vi "Progress bar v2.vi"(7 "TIme (s)":dbl=10.0, 8 "error in":errorcluster, 11 "Title":string="Preparing GUI") -> (0 "error out":errorcluster)   [LabVIEW 2021]
uses:
  <vilib>/NI/Progress Bar/Controls/Update Bar Actions.ctl
  <vilib>/NI/Progress Bar/Controls/Progress Bar Properties.ctl
  f8578292-8b37-437c-93d2-4d8660ecfccc.vi
  114d9f00-15c4-4ec7-b9fc-572f42474f64.vi
  911e5ed0-5c28-4744-8a2b-9f7e262dfa91.vi
  eb646fbe-3ace-4864-911c-cb9f93faacb5.vi
  875ffc95-6fd8-47bf-be2f-a53a9a05b130.vi
  8d024e92-ce25-45d8-b0eb-876bcb212ffe.vi
  0a453649-e7a0-4eaf-b47a-dfd7043e0d01.vi
  be3f16ba-4c0f-4040-8c78-39f5a151251f.vi
  12f81415-701e-4c93-8868-a36497b1982f.vi
  <vilib>/NI/Progress Bar/Progress Bar.lvlib
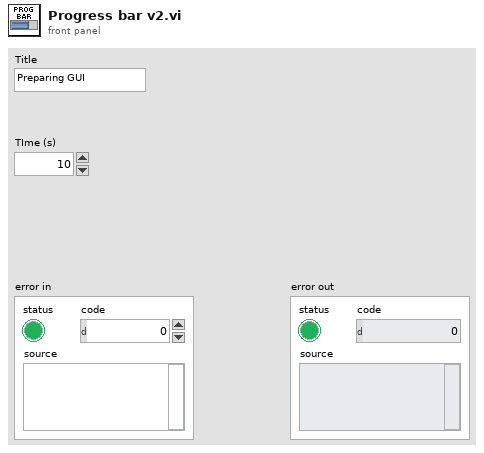
[diagram p1: front panel]
types:
  T1 = typedef "Progress Bar.lvlib/Progress Bar Properties.ctl" = cluster{"Background Color":u32, "Installer Title":string, "Title Color":u32, "Action Text":string, "Text Color":u32, "Slider Value":u8, "Bar Color":u32, "Timeout":i32}
  T2 = typedef "Progress Bar.lvlib/Update Bar Actions.ctl" = enum16{"Add To Existing", "Set to Value"}
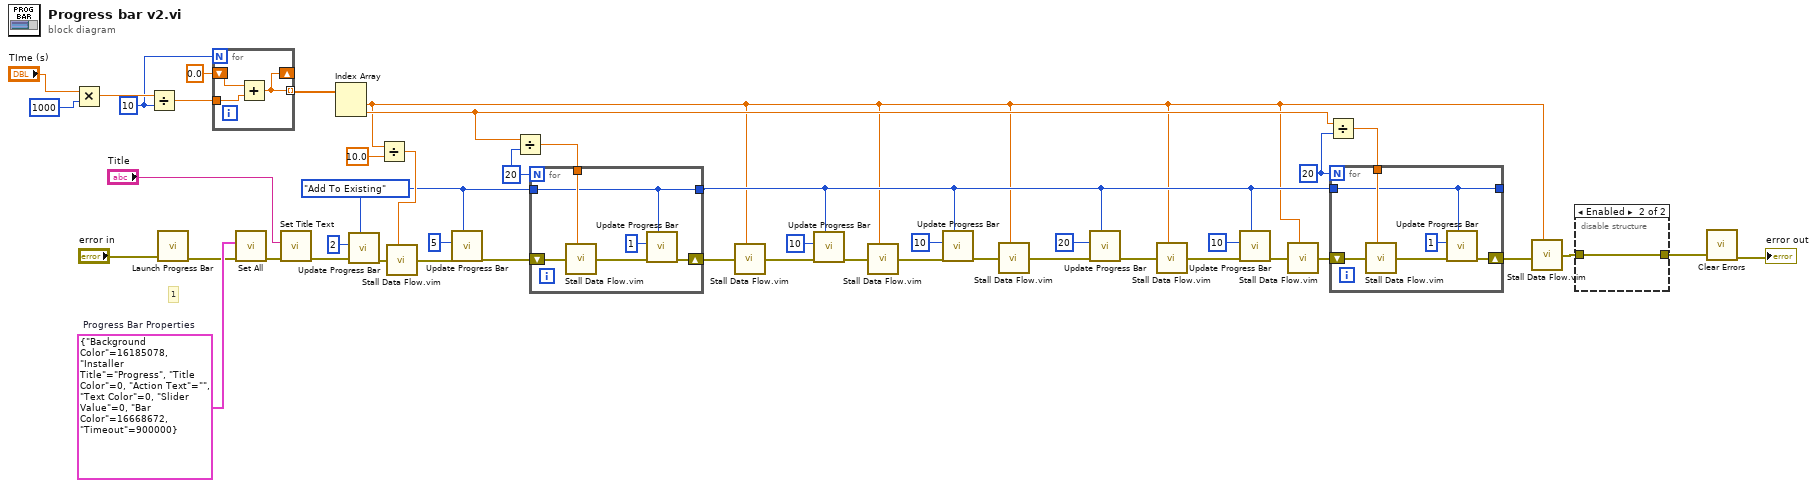
[diagram p0: block diagram]
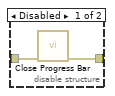
[diagram p2: hidden frame]
diagram:
  w11 = 20
  w32 = u32 10 ("y")
  w41 = T1 {"Background Color"=16185078, "Installer Title"="Progress", "Title Color"=0, "Action Text"="", "Text Color"=0, "Slider Value"=0, "Bar Color"=16668672, "Timeout"=900000}  # Progress Bar Properties
  w27 = 20 ("Value")
  w9 = Update_Bar_Actions."Add To Existing" ("Action")
  # "1"
  n1 = Multiply(x="TIme (s)", y=1000) -> (x*y=w33:dbl)
  n2 = Divide(x=w33, y=w32) -> (x/y=w31:dbl)
  n3 = call <vilib>:"Launch Progress Bar.vi"("error in (no error)"="error in") -> ("error out"=w37:errorcluster)  [unwired: 9 in, 1 out]
  n4 = for {
    N: w32 -> [_]
    shift-right: [w47] -> _
    shift-left: 0.0 -> [w49]
    tunnel: w31 -> [w48]
    tunnel: [w47] -> w30 mode=indexing
    n5 = Add(x=w49, y=w48) -> (x+y=w47:dbl)
  }
  n6 = call <vilib>:"Set All.vi"("error in (no error)"=w37, "Progress Bar Properties (Default)"=w41) -> ("error out"=w45:errorcluster)  [unwired: 9 in]
  n7 = call <vilib>:"Set Title Text.vi"("error in (no error)"=w45, "Installer Title"="Title") -> ("error out"=w20:errorcluster)  [unwired: 9 in]
  n8 = Index Array(array=w30) -> (element #1=w3:dbl, element #2=w5:dbl)  [unwired: 2 in]
  n9 = call <vilib>:"Update Progress Bar.vi"("Action"=w9, "error in (no error)"=w20, "Value"=u8 2) -> ("error out"=w19:errorcluster)  [unwired: 8 in]
  n10 = Divide(x=w3, y=10.0) -> (x/y=w16:dbl)
  n11 = call "Stall Data Flow.vim"("value in"=w19, "milliseconds to wait"=w16) -> ("value out"=w17:errorcluster)  [unwired: 1 out]
  n12 = call <vilib>:"Update Progress Bar.vi"("Action"=w9, "error in (no error)"=w17, "Value"=u8 5) -> ("error out"=w13:errorcluster)  [unwired: 8 in]
  n13 = Divide(x=w5, y=w11) -> (x/y=w10:dbl)
  n14 = for {
    N: w11 -> [_]
    tunnel: w9 -> [w50]
    shift-right: [w55] -> w12
    shift-left: w13 -> [w54]
    tunnel: w10 -> [w51]
    tunnel: [w50] -> w8
    n15 = call "Stall Data Flow.vim"("value in"=w54, "milliseconds to wait"=w51) -> ("value out"=w52:errorcluster)  [unwired: 1 out]
    n16 = call <vilib>:"Update Progress Bar.vi"("Action"=w50, "error in (no error)"=w52, "Value"=u8 1) -> ("error out"=w55:errorcluster)  [unwired: 8 in]
  }
  n17 = call "Stall Data Flow.vim"("value in"=w12, "milliseconds to wait"=w3) -> ("value out"=w7:errorcluster)  [unwired: 1 out]
  n18 = call <vilib>:"Update Progress Bar.vi"("Action"=w8, "error in (no error)"=w7, "Value"=u8 10) -> ("error out"=w15:errorcluster)  [unwired: 8 in]
  n19 = call "Stall Data Flow.vim"("value in"=w15, "milliseconds to wait"=w3) -> ("value out"=w6:errorcluster)  [unwired: 1 out]
  n20 = call <vilib>:"Update Progress Bar.vi"("Action"=w8, "error in (no error)"=w6, "Value"=u8 10) -> ("error out"=w39:errorcluster)  [unwired: 8 in]
  n21 = call "Stall Data Flow.vim"("value in"=w39, "milliseconds to wait"=w3) -> ("value out"=w29:errorcluster)  [unwired: 1 out]
  n22 = call <vilib>:"Update Progress Bar.vi"("Action"=w8, "error in (no error)"=w29, "Value"=u8 20) -> ("error out"=w38:errorcluster)  [unwired: 8 in]
  n23 = call "Stall Data Flow.vim"("value in"=w38, "milliseconds to wait"=w3) -> ("value out"=w28:errorcluster)  [unwired: 1 out]
  n24 = call <vilib>:"Update Progress Bar.vi"("Action"=w8, "error in (no error)"=w28, "Value"=u8 10) -> ("error out"=w40:errorcluster)  [unwired: 8 in]
  n25 = call "Stall Data Flow.vim"("value in"=w40, "milliseconds to wait"=w3) -> ("value out"=w25:errorcluster)  [unwired: 1 out]
  n26 = Divide(x=w5, y=w27) -> (x/y=w26:dbl)
  n27 = for {
    N: w27 -> [_]
    tunnel: w8 -> [w56]
    shift-right: [w61] -> w24
    shift-left: w25 -> [w60]
    tunnel: w26 -> [w57]
    tunnel: [w56] -> _
    n28 = call "Stall Data Flow.vim"("value in"=w60, "milliseconds to wait"=w57) -> ("value out"=w58:errorcluster)  [unwired: 1 out]
    n29 = call <vilib>:"Update Progress Bar.vi"("Action"=w56, "error in (no error)"=w58, "Value"=u8 1) -> ("error out"=w61:errorcluster)  [unwired: 8 in]
  }
  n30 = call "Stall Data Flow.vim"("value in"=w24, "milliseconds to wait"=w3) -> ("value out"=w22:errorcluster)  [unwired: 1 out]
  n31 = disable-structure shown="Enabled" {
    disable-tunnel: w22 -> [w63 w64]
    disable-tunnel: [w62 w64] -> w2
    frame Disabled {
      n32 = call <vilib>:"Close Progress Bar.vi"("error in (no error)"=w63) -> ("error out"=w62:errorcluster)  [unwired: 9 in, 1 out]
    }
    frame Enabled {
    }
  }
  n33 = call <vilib>:"Clear Errors.vi"("error in (no error)"=w2) -> ("error out"=→"error out":errorcluster)  [unwired: 5 in, 1 out]
